vi "Station Report Errors.vi"(8 "error in (no error)":errorcluster) -> (0 "error out":errorcluster)   [LabVIEW 2018, in "Station.lvclass"]
uses:
  Station.lvclass
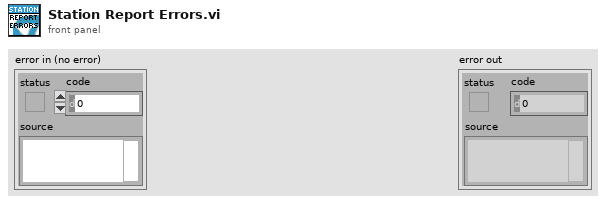
[diagram p1: front panel]
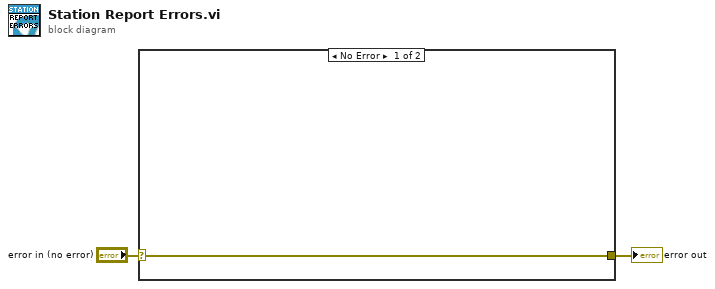
[diagram p0: block diagram]
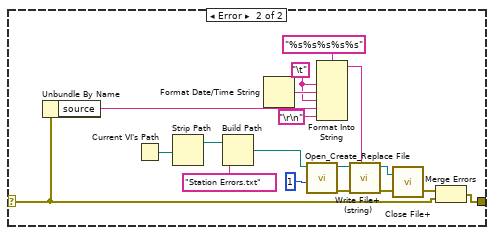
[diagram p2: hidden frame]
diagram:
  n1 = case shown="No Error" "error in (no error)" {
    selector: "error in (no error)" -> [w3 w10]
    tunnel: [w3 w11] -> w1
    frame No Error {
    }
    frame Error {
      w13 = "\t"
      n2 = Unbundle By Name(w10) -> ("source"=w9:string)
      n3 = Current VI's Path() -> (path=w7:path)
      n4 = Strip Path(path=w7) -> (stripped path=w6:path)  [unwired: 1 out]
      n5 = Build Path(base path=w6, name or relative path="Station Errors.txt") -> (appended path=w4:path)
      n6 = Format Date/Time String() -> (date/time string=w14:string)  [unwired: 3 in]
      n7 = call <vilib>:"Open_Create_Replace File.vi"("function (open:0)"=1, "file path"=w4) -> ("error out"=w18:errorcluster, "refnum"=w20:refnum<file>)  [unwired: 6 in, 2 out]
      n8 = Format Into String(format string="%s%s%s%s%s", w13, w14, w13, w9, "\r\n") -> (resulting string=w12:string)  [unwired: 2 in, 1 out]
      n9 = call <vilib>:"Write File+ (string).vi"("string"=w12, "error in (no error)"=w18, "refnum"=w20) -> ("error out"=w17:errorcluster, "dup refnum"=w21:refnum<file>)  [unwired: 4 in, 1 out]
      n10 = call <vilib>:"Close File+.vi"("error in (no error)"=w17, "refnum"=w21) -> ("error out"=w16:errorcluster)  [unwired: 3 in, 2 out]
      n11 = Merge Errors(w16, w10) -> (w11:errorcluster)
    }
  }
  "error out" <- w1
